vi "_MT_Init.vi"(8 "Error In":errorcluster) -> (0 "Error Out":errorcluster)   [LabVIEW 2020, in "MT_API.lvlib"]
doc: "MT_API INT32 __stdcall MT_Init(void);"
uses:
  MT_API.lvlib
  MT_API_64.dll
panel:
  out "函数返回值":i32
  # "初始化MT设备的相关资源"
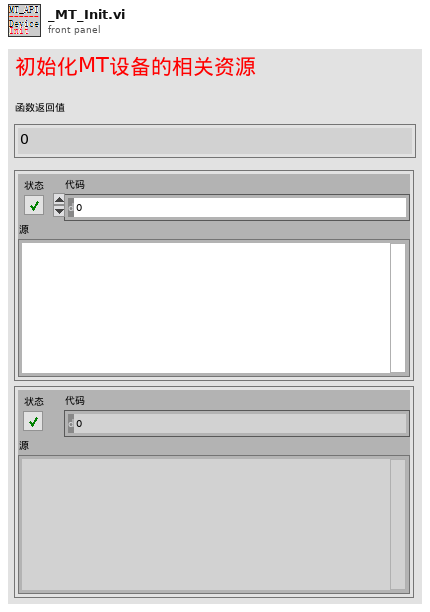
[diagram p1: front panel]
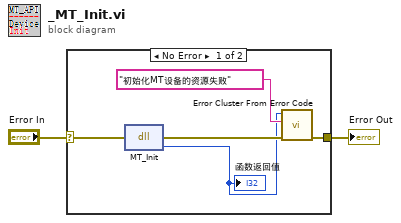
[diagram p0: block diagram]
diagram:
  n1 = case shown="No Error" "Error In" {
    selector: "Error In" -> [w7 w8]
    tunnel: [w3 w8] -> w1
    frame No Error {
      n2 = dll-call lib="D:/Project NJU/lib/MT/MT_API_64.*" fn="MT_Init"(error in=w7) -> (error out=w6:errorcluster, "return type"=w4:i32)  [unwired: 2 in, 1 out]
      "函数返回值" <- w4
      n3 = call <vilib>:"Error Cluster From Error Code.vi"("error in (no error)"=w6, "error message (\"\")"="初始化MT设备的资源失败", "error code (0)"=w4) -> ("error out"=w3:errorcluster)  [unwired: 6 in]
    }
    frame Error {
    }
  }
  "Error Out" <- w1
